vi "Cholesky Factorization Rank-1 Update_Downdate (CDB).vi"(10 "X":cdb[](array[numeric]), 11 "R":T1) -> (0 "error":i32, 3 "Updated R":T1)   [LabVIEW 2017, in "NI_AAL_LinAlg.lvlib"]
uses:
  <vilib>/Analysis/NI_AAL_LinAlg.lvlib
  <vilib>/Analysis/Matrix/Datatypes/ComplexMatrix.ctl
  <vilib>/Analysis/baseanly.llb/Matrix Type of Inverse Matrix.ctl
  <vilib>/Analysis/7linalg.llb/Complex Conjugate Transpose Matrix.vi
  <vilib>/Analysis/baseanly.llb/Unit Vector (CDB).vi
  <vilib>/Analysis/7linalg.llb/Solve Complex Linear Equations (single right hand).vi
  <vilib>/Analysis/NI_AALBase.lvlib
  <vilib>/Analysis/NI_AALPro.lvlib
  <vilib>/Analysis/Matrix/NI_Matrix.lvlib
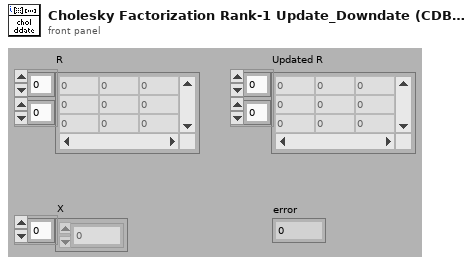
[diagram p1: front panel]
types:
  T1 = typedef "NI_Matrix.lvlib/ComplexMatrix.ctl" = cdb[][]
  T2 = typedef "NI_AALBase.lvlib/Matrix Type of Inverse Matrix.ctl" = enum32{"General", "Positive Definite", "Lower Triangular", "Upper Triangular"}
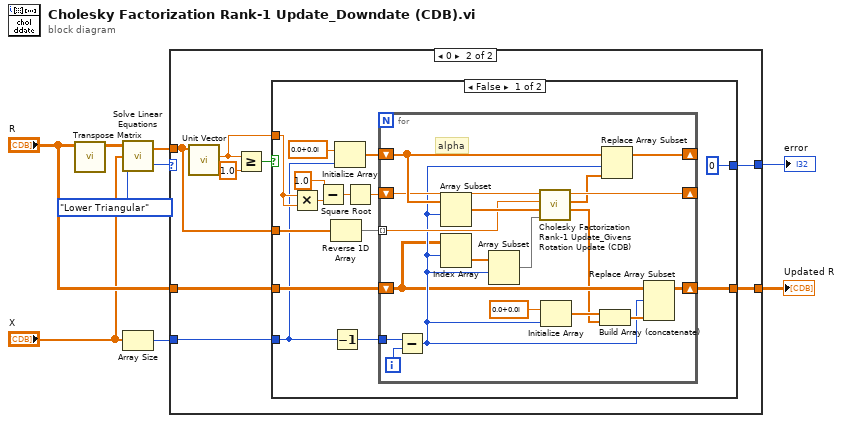
[diagram p0: block diagram]
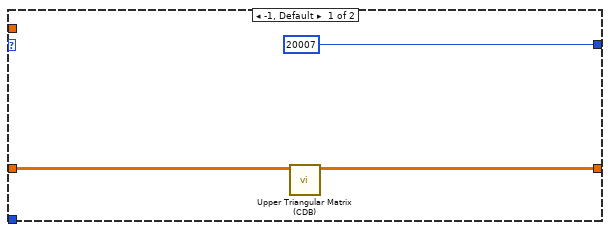
[diagram p2: hidden frame]
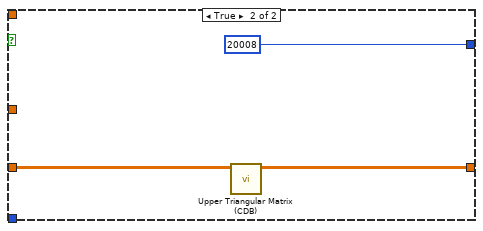
[diagram p3: hidden frame]
diagram:
  n1 = call-poly <vilib>:"Transpose Matrix.vi"("Input Matrix"="R") -> ("Matrix Conjugate Transpose"=w5:T1)  [unwired: 9 in, 1 out]
  n2 = call-poly <vilib>:"Solve Linear Equations.vi"("matrix type"=Matrix_Type_of_Inverse_Matrix."Lower Triangular", "Known Vector"="X", "Input Matrix"=w5) -> ("error"=w7:i32, "Solution Vector"=w8:cdb[])
  n3 = Array Size(array="X") -> (size(s)=w9:i32)
  n4 = case shown="0" w7 {
    tunnel: w8 -> [_ w14]
    tunnel: "R" -> [w10 w15]
    tunnel: [w11 w18] -> w2
    tunnel: [20007 w17] -> w1
    tunnel: w9 -> [_ w16]
    frame -1, Default {
      n5 = call <vilib>:"Upper Triangular Matrix (CDB).vi"("A"=w10) -> ("U"=w11:T1)  [unwired: 10 in]
    }
    frame 0 {
      n6 = call-poly <vilib>:"Unit Vector.vi"("Input Vector"=w14) -> ("norm"=w13:dbl)  [unwired: 2 in, 8 out]
      n7 = Greater Or Equal?(x=w13, y=1.0) -> (x >= y?=w19:bool)
      n8 = case shown="False" w19 {
        tunnel: w14 -> [w30 _]
        tunnel: w13 -> [w34 _]
        tunnel: w15 -> [w28 w53]
        tunnel: [w22 w54] -> w18
        tunnel: [0 20008] -> w17
        tunnel: w16 -> [w24 _]
        frame False {
          n9 = Multiply(x=w34, y=w34) -> (x*y=w33:dbl)
          n10 = Subtract(x=1.0, y=w33) -> (x-y=w26:dbl)
          n11 = Reverse 1D Array(array=w30) -> (reversed array=w23:cdb[])
          n12 = Decrement(x=w24) -> (x-1=w31:i32)
          n13 = Initialize Array(cdb 0.0+0.0i ("x+y"), w24) -> (w29:cdb[])
          n14 = Square Root(x=w26) -> (sqrt(x)=w25:dbl)
          n15 = for {
            shift-right: [w38] -> _
            shift-left: w25 -> [w46]
            tunnel: w31 -> [w52]
            tunnel: w23 -> [w43] mode=indexing
            shift-right: [w49] -> _
            shift-left: w29 -> [w50]
            shift-right: [w39] -> w22
            shift-left: w28 -> [w40]
            i -> [w51]
            # "alpha"
            n16 = Subtract(x=w52, y=w51) -> (x-y=w41:i32)
            n17 = Array Subset(array=w50, index=w41) -> (w45:cdb[])  [unwired: 1 in]
            n18 = Index Array(array=w40, index (row)=w41) -> (element=w47:cdb[])  [unwired: 1 in]
            n19 = Array Subset(array=w47, index=w41) -> (w44:cdb[])  [unwired: 1 in]
            n20 = call <vilib>:"Cholesky Factorization Rank-1 Update_Givens Rotation Update (CDB).vi"("Y In"=w44, "X In"=w45, "b"=w43, "a"=w46) -> ("Y Out"=w35:cdb[], "X Out"=w36:cdb[], "v"=w38:cdb)  [unwired: 5 in]
            n21 = Initialize Array(cdb 0.0+0.0i ("element"), w41) -> (w48:cdb[])
            n22 = Build Array (concatenate)(w48, w35) -> (w42:cdb[])
            n23 = Replace Array Subset(array=w50, new element=w36, index=w41) -> (w49:cdb[])
            n24 = Replace Array Subset(array=w40, new element=w42, index (row)=w41) -> (w39:T1)  [unwired: 1 in]
          }
        }
        frame True {
          n25 = call <vilib>:"Upper Triangular Matrix (CDB).vi"("A"=w53) -> ("U"=w54:T1)  [unwired: 10 in]
        }
      }
    }
  }
  "Updated R" <- w2
  "error" <- w1
